vi "Cryo-Con Get Settigns.vi"(8 "Error In":errorcluster, 10 "Inputs":string[](array[string]), 11 "VISA resource name":refnum<visa-resource-name>) -> (0 "Error Out":errorcluster, 1 "Settings":string, 3 "VISA resource name out":refnum<visa-resource-name>)   [LabVIEW 2019]
uses:
  GPIB/VISA  Send Receive.vi
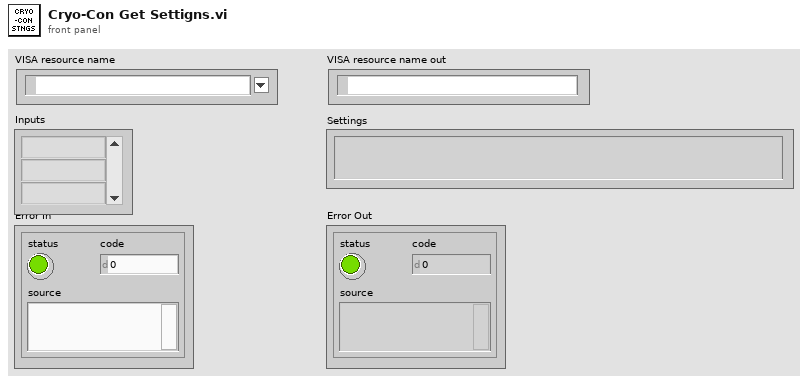
[diagram p1: front panel]
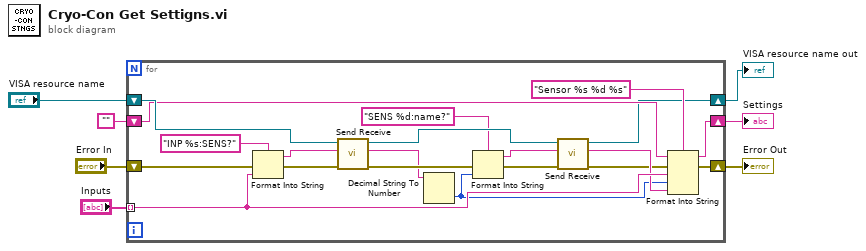
[diagram p0: block diagram]
diagram:
  n1 = for {
    shift-right: [w11] -> w3
    shift-left: "VISA resource name" -> [w27]
    shift-right: [w22] -> w4
    shift-left: "Error In" -> [w24]
    tunnel: "Inputs" -> [w20] mode=indexing
    shift-right: [w19] -> w5
    shift-left: "" -> [w18]
    n2 = Format Into String(format string="INP %s:SENS?", error in=w24, w20) -> (resulting string=w25:string, error out=w23:errorcluster)  [unwired: 1 in]
    n3 = call-poly "Send Receive.vi"("error in (no error)"=w23, "data string in"=w25, "VISA Resource Name"=w27) -> ("error out"=w16:errorcluster, "data string out"=w13:string, "VISA Resource Name Out"=w17:refnum<visa-resource-name>)  [unwired: 6 in]
    n4 = Decimal String To Number(string=w13) -> (number=w8:i32)  [unwired: 2 in, 1 out]
    n5 = Format Into String(format string="SENS %d:name?", error in=w16, w8) -> (resulting string=w9:string, error out=w15:errorcluster)  [unwired: 1 in]
    n6 = call-poly "Send Receive.vi"("error in (no error)"=w15, "data string in"=w9, "VISA Resource Name"=w17) -> ("error out"=w10:errorcluster, "data string out"=w12:string, "VISA Resource Name Out"=w11:refnum<visa-resource-name>)  [unwired: 6 in]
    n7 = Format Into String(format string="Sensor %s %d %s", initial string=w18, error in=w10, w20, w8, w12) -> (resulting string=w19:string, error out=w22:errorcluster)
  }
  "VISA resource name out" <- w3
  "Error Out" <- w4
  "Settings" <- w5
